vi "Queue's FGV.vi"(11 "error in":errorcluster, 13 "Create new?":bool) -> (4 "Cluster":cluster{"DO-Interupt-Q":refnum<queue>}, 15 "error out":errorcluster)   [LabVIEW 2021]
uses:
  TCP Engine/Controls/TCP Engine I&O  Interupt Cluster.ctl
  Controls/RT-ALl Queue Name's.ctl
  98d8c211-cb34-4886-8f40-5d90e9bde849.vi
  TCP Engine/TCP Engine.lvlib
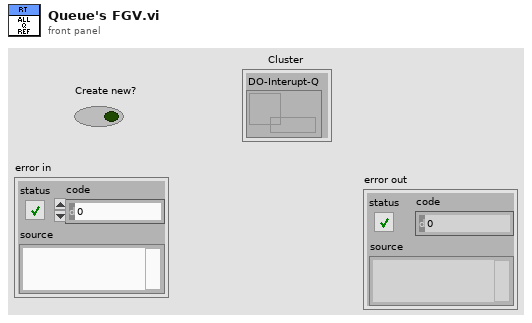
[diagram p1: front panel]
types:
  T1 = typedef "RT-ALl Queue Name's.ctl" = enum16{"DO-Interupt Q"}
  T2 = typedef "TCP Engine.lvlib/TCP Engine I&O  Interupt Cluster.ctl" = cluster{" Stop":bool, "JSON Variant":variant}
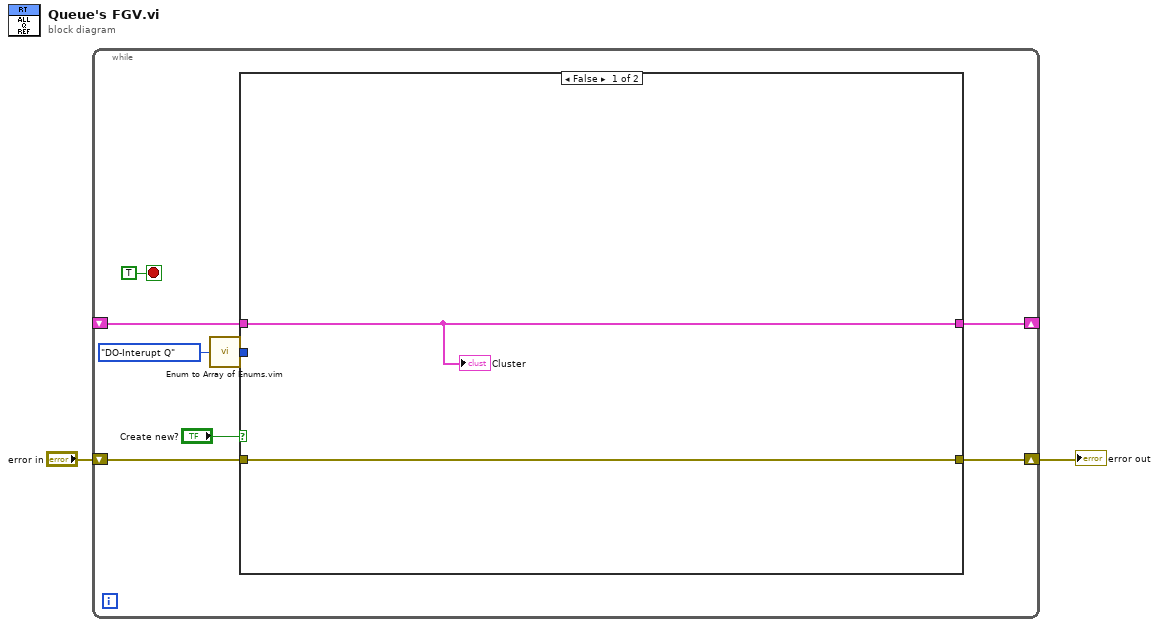
[diagram p0: block diagram]
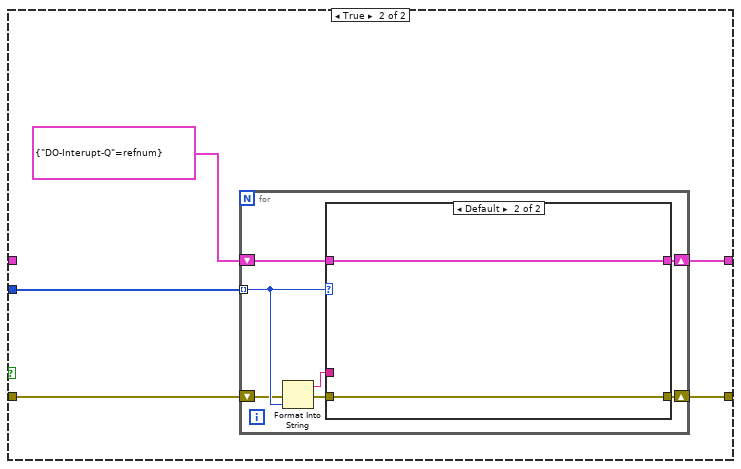
[diagram p2: hidden frame]
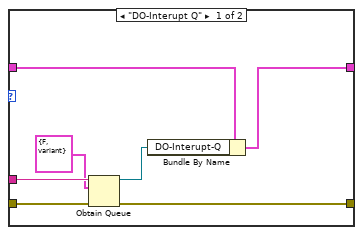
[diagram p3: hidden frame]
diagram:
  n1 = while {
    shift-right: [w10] -> w2
    shift-left: "error in" -> [w9]
    shift-right: [w7] -> _
    shift-left: _ -> [w6]
    stop <- TRUE stop-if-true
    n2 = call "Enum to Array of Enums.vim"("enum"=RT-ALl_Queue_Name's."DO-Interupt Q" ("All-Queue Name's")) -> ("array of enums"=w4:T1[])
    n3 = case shown="False" "Create new?" {
      tunnel: [w12 w16] -> w10
      tunnel: w9 -> [w12 w17]
      tunnel: [w11 w13] -> w7
      tunnel: w6 -> [w11 _]
      tunnel: w4 -> [_ w15]
      frame False {
        "Cluster" <- w11
      }
      frame True {
        n4 = for {
          shift-right: [w24] -> w16
          shift-left: w17 -> [w21]
          tunnel: w15 -> [w23] mode=indexing
          shift-right: [w19] -> w13
          shift-left: cluster{"DO-Interupt-Q":refnum<queue>} {"DO-Interupt-Q"=refnum} -> [w18]
          n5 = Format Into String(error in=w21, w23) -> (resulting string=w22:string, error out=w20:errorcluster)  [unwired: 2 in]
          n6 = case shown="Default" w23 {
            tunnel: w20 -> [w31 w33]
            tunnel: [w30 w33] -> w24
            tunnel: w22 -> [w29 _]
            tunnel: [w25 w32] -> w19
            tunnel: w18 -> [w27 w32]
            frame "DO-Interupt Q" {
              n7 = Obtain Queue(name (unnamed)=w29, element data type=T2 {" Stop"=FALSE, "JSON Variant"=variant(string "")} ("I/O  Interupt Cluster"), error in (no error)=w31) -> (queue out=w26:refnum<queue>, error out=w30:errorcluster)  [unwired: 2 in, 1 out]
              n8 = Bundle By Name(cluster=w27, "DO-Interupt-Q"=w26) -> (w25:cluster{"DO-Interupt-Q":refnum<queue>})
            }
            frame Default {
            }
          }
        }
      }
    }
  }
  "error out" <- w2
